vi "Delievery.vi"() -> ()   [LabVIEW 2016]
panel:
  in  "Previous Button":bool
  # "Kounotori (HTV)"
  # "Delivery"
  # "Dragon (SpaceX)"
  # "Unmanned spaceflights to the International Space Station (ISS) are made primarily to deliver cargo, however several Russian modules have also docked to the outpost following unmanned launches. Resupply missions typically use the Russian Progress spacecraft, European Automated Transfer Vehicles, Japanese Kounotori vehicles, and the American Dragon and Cygnus spacecraft. The primary docking system for Progress spacecraft is the automated Kurs system, with the manual TORU system as a backup. ATVs also use Kurs, however they are not equipped with TORU. Progress and ATV can remain docked for up to six months.The other spacecraft — the Japanese HTV, the SpaceX Dragon and the Orbital Sciences Cygnus — rendezvous with the station before being grappled using Canadarm2 and berthed at the nadir port of the Harmony or Unity module for one to two months. As of March 2017, Progress spacecraft have flown most of the unmanned missions to the ISS."
  # "Cygnus"
  # "Progress Supply Ship"
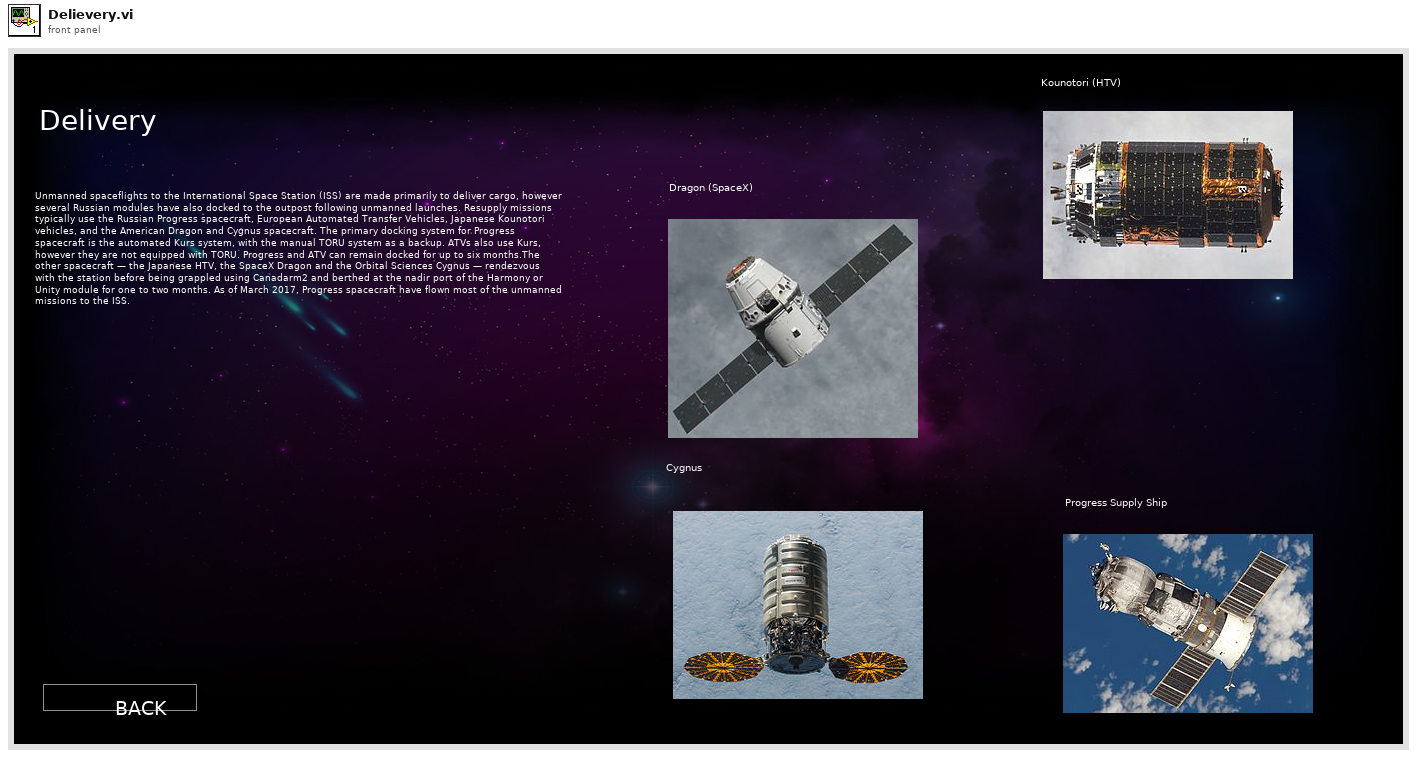
[diagram p1: front panel]
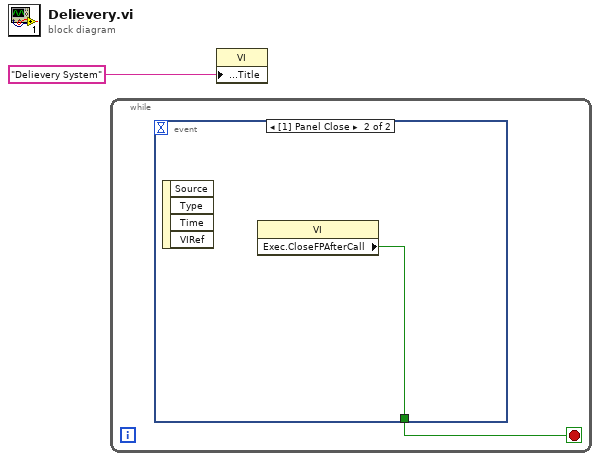
[diagram p0: block diagram]
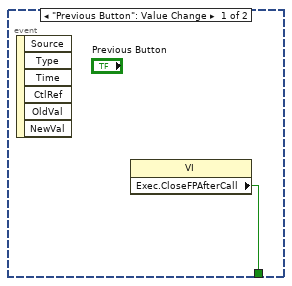
[diagram p2: hidden frame]
diagram:
  n1 = while {
    stop <- w2 stop-if-true
    n2 = event shown="[1] Panel Close" {
      selector: _ -> [_ _]
      dyn-events: _ -> [_ _]
      timeout: _ -> [_ _]
      tunnel: [w3 w4] -> w2
      event "Previous Button": Value Change {
        n3 = event-data() -> ()  [unwired: 1 in, 6 out]
        n4 = property class="VI"() -> ("Exec.CloseFPAfterCall"=w3:bool)  [unwired: 2 in, 2 out]
      }
      event Panel Close {
        n5 = event-data() -> ()  [unwired: 1 in, 4 out]
        n6 = property class="VI"() -> ("Exec.CloseFPAfterCall"=w4:bool)  [unwired: 2 in, 2 out]
      }
    }
  }
  n7 = property class="VI"("Front Panel.Title"="Delievery System" ("Front Panel Window:Title")) -> ()  [unwired: 2 in, 2 out]
